vi "Read Copy Data.vi"(8 "error in (no error)":errorcluster) -> (0 "error out":errorcluster, 3 "xml string":string)   [LabVIEW 2021]
uses:
  <userlib>/John_Lib/TopPath/TopPath.lvlib
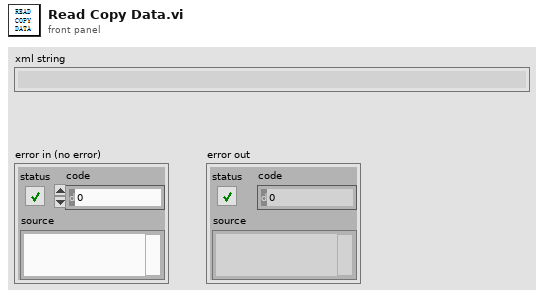
[diagram p1: front panel]
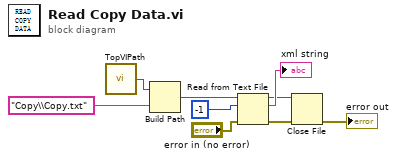
[diagram p0: block diagram]
diagram:
  n1 = call <userlib>:"TopVIPath.vi"() -> ("ConfigFile path"=w6:path)  [unwired: 2 out]
  n2 = Build Path(base path=w6, name or relative path="Copy\\Copy.txt" ("xml string")) -> (appended path=w7:path)
  n3 = Read from Text File(file (use dialog)=w7, count=-1, error in="error in (no error)") -> (refnum out=w3:refnum<file>, text=→"xml string":string, error out=w2:errorcluster)  [unwired: 1 in, 1 out]
  n4 = Close File(refnum=w3, error in=w2) -> (error out=→"error out":errorcluster)  [unwired: 1 out]
